vi "test_ThreeSessTwoPinThreeInstrTwoSiteReservation_CallNiDmmGetConnections1Pin1Connection_ReturnsOneConnection.vi"(8 "error in":errorcluster) -> (0 "error out":errorcluster, 2 "result":string, 3 "pass":bool)   [LabVIEW 2020, in "MeasurementServerTests.lvlib"]
uses:
  MeasurementServerTests.lvlib
  Runtime/Clients/Session Management V1/Session Reservation/Connection.ctl
  Runtime/Clients/Session Management V1/Session Reservation/Session Reservation.lvclass
  03fc85e1-696b-4ece-a78b-f41470766ac0.vi
  Runtime/Sessions/niDMM/Connection with Session.ctl
  Runtime/Sessions/niDMM/NI Session Management niDMM.lvlib
  c6c17ed5-74bf-42ea-8308-b396c43a9178.vi
  Runtime/Sessions/niDMM/Get Connections - 1Pin 1Conn.vi
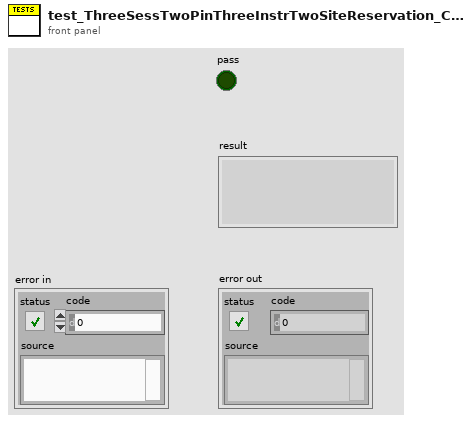
[diagram p1: front panel]
types:
  T1 = typedef "NI Session Management niDMM.lvlib/Connection with Session.ctl" = cluster{"connection":T2, "session":refnum<k15>}
  T2 = typedef "NI Session Management V1 Client.lvlib/Session Reservation.lvclass/Connection.ctl" = cluster{"pin or relay name":string, "site":i32, "instrument type id":string, "channel":string}
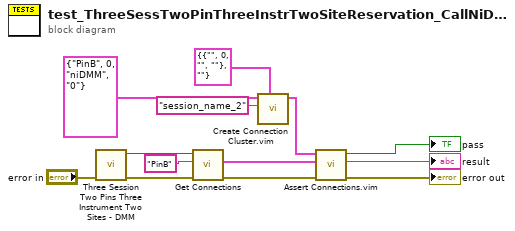
[diagram p0: block diagram]
diagram:
  n1 = call "Three Session Two Pins Three Instrument Two Sites - DMM.vi"("error in"="error in") -> ("error out"=w3:errorcluster, "session reservation out"=w4:refnum<class "Session Reservation.lvclass">)  [unwired: 9 in]
  n2 = call-poly "Get Connections.vi"("error in"=w3, "pin or relay name"="PinB", "session reservation in"=w4) -> ("error out"=w2:errorcluster, "connection"=w7:T1)  [unwired: 6 in, 1 out]
  n3 = call "Create Connection Cluster.vim"("connection type"=T1 {"connection"={"pin or relay name"="", "site"=0, "instrument type id"="", "channel"=""}, "session"=""} ("connection with session"), "session in"="session_name_2", "hardware independent connection in"=T2 {"pin or relay name"="PinB", "site"=0, "instrument type id"="niDMM", "channel"="0"} ("connection")) -> ("connection out"=w11:T1)  [unwired: 8 in]
  n4 = call "Assert Connections.vim"("error in"=w2, "actual connections"=w7, "expected connections"=w11) -> ("error out"=→"error out":errorcluster, "result"=→"result":string, "pass"=→"pass":bool)  [unwired: 6 in]
